vi "校准设置页.vi"() -> ()   [LabVIEW 2016, in "斯坦道总氮V2.lvlib"]
uses:
  <vilib>/regexp/Match Regular Expression.xnode
  <vilib>/ptbypt/NI_PtbyPt.lvlib
panel:
  in  "校准任务":bool
  in  "历史数据导入":T1(radio)
  out "刷新时间":string
  out "模型刷新":bool
  in  "校准按钮":T1(radio)
  in  "仪器写入":bool
  in  "辅助计算":bool
  in  "曲线模型":T2={"标液浓度1"=0.0, "测量吸光度1"=0.0, "样品1启用"=FALSE, "标液浓度2"=0.0, "测量吸光度2"=0.0, "样品2启用"=FALSE, "标液浓度3"=0.0, "测量吸光度3"=0.0, "样品3启用"=FALSE, "标液浓度4"=0.0, "测量吸光度4"=0.0, "样品4启用"=FALSE, "标液浓度5"=0.0, "测量吸光度5"=0.0, "样品5启用"=FALSE, "模型"=enum."线性", "精度"=4.0, "XY图"=[], "拟合公式"="", "r^2"=0.0, "标样一校准时间"=timestamp(0 s since 1904-01-01), "标样二校准时间"=timestamp(0 s since 1904-01-01), "标样三校准时间"=timestamp(0 s since 1904-01-01), "标样四校准时间"=timestamp(0 s since 1904-01-01), "标样五校准时间"=timestamp(0 s since 1904-01-01), "二次方程"={"c"=0.0, "x"=0.0, "x^2"=0.0}, "标定时间"=timestamp(0 s since 1904-01-01)} {"标定时间" format="%<%y/%m/%d %H:%M:%S>T"; "标样五校准时间" format="%<%y/%m/%d %H:%M:%S>T"; "标样四校准时间" format="%<%y/%m/%d %H:%M:%S>T"; "标样三校准时间" format="%<%y/%m/%d %H:%M:%S>T"; "标样二校准时间" format="%<%y/%m/%d %H:%M:%S>T"; "标样一校准时间" format="%<%y/%m/%d %H:%M:%S>T"; "r^2" format="%.7f"; "测量吸光度5" format="%#.6f"; "测量吸光度4" format="%#.6f"; "测量吸光度3" format="%#.6f"; "测量吸光度2" format="%#.6f"; "测量吸光度1" format="%#.6f"}
  in  "测量模式":enum16{"跨度核查", "水样测量", "零点核查", "标样核查", "加标回收"}(ring)
  in  "参数下拉列表":u16(ring)
  in  "量程下拉列表":enum16{"低量程", "高量程"}(ring)
  # "校准时间"
  # "标液浓度"
  # "吸光值"
  # "标样一"
  # "标样二"
  # "标样三"
  # "零点"
  # "跨度"
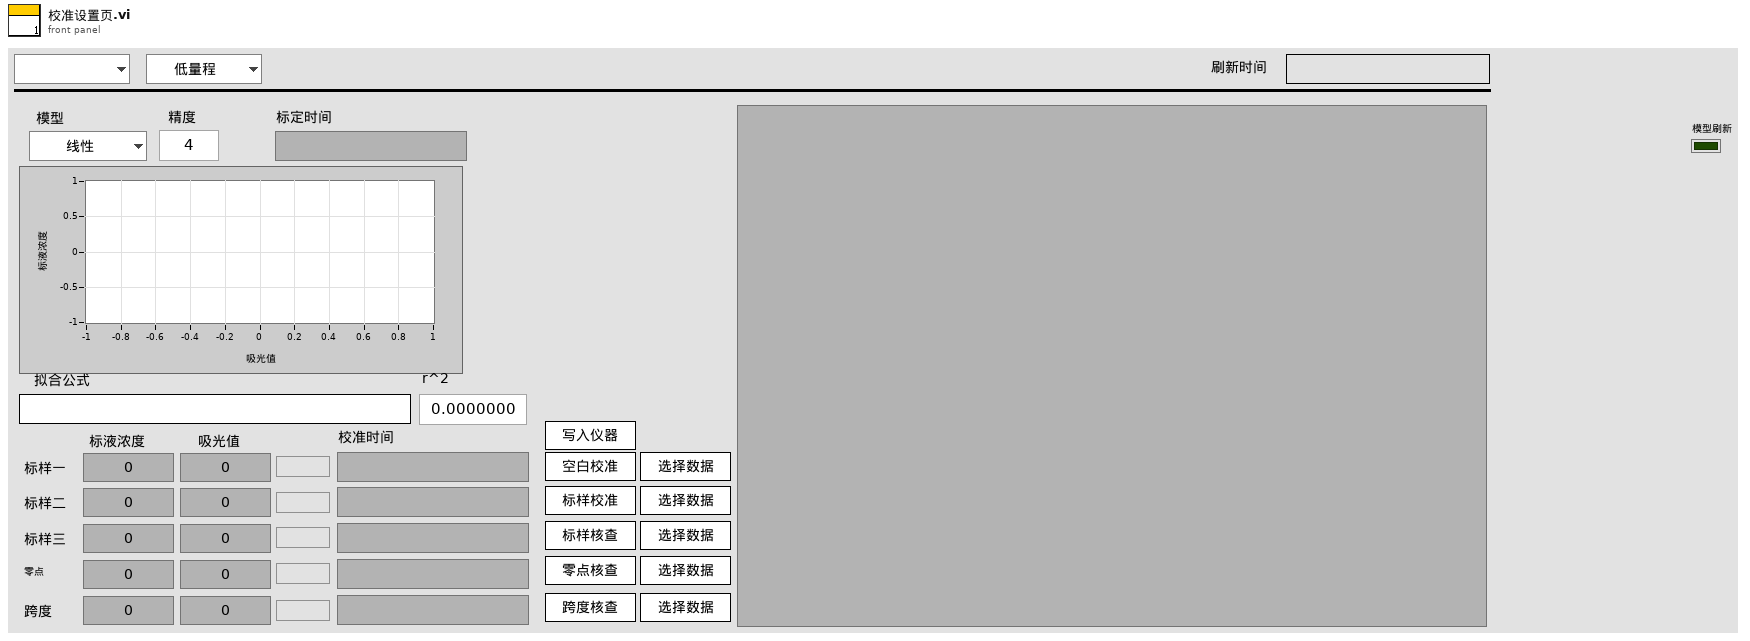
[diagram p1: front panel]
types:
  T1 = enum32{"未选择", "空白校准", "标样校准", "标样核查", "零点核查", "跨度核查"}
  T2 = cluster{"标液浓度1":dbl, "测量吸光度1":dbl, "样品1启用":bool, "标液浓度2":dbl, "测量吸光度2":dbl, "样品2启用":bool, "标液浓度3":dbl, "测量吸光度3":dbl, "样品3启用":bool, "标液浓度4":dbl, "测量吸光度4":dbl, "样品4启用":bool, "标液浓度5":dbl, "测量吸光度5":dbl, "样品5启用":bool, "模型":enum32{"线性", "多项式"}, "精度":dbl, "XY图":cluster{"X Values":dbl[], "Y Values":dbl[]}[], "拟合公式":string, "r^2":dbl, "标样一校准时间":timestamp, "标样二校准时间":timestamp, "标样三校准时间":timestamp, "标样四校准时间":timestamp, "标样五校准时间":timestamp, "二次方程":cluster{"c":dbl, "x":dbl, "x^2":dbl}, "标定时间":timestamp}
  T3 = typedef "斯坦道总氮V2.lvlib/校准任务.ctl" = cluster{"id":u16, "任务类型":enum16{"未选择", "空白校准", "标样校准", "标样核查", "零点核查", "跨度核查"}, "量程下拉列表":enum16{"低量程", "高量程"}, "状态":enum16{"已执行", "待执行", "执行中", "停止"}, "标液浓度":dbl, "吸光值":dbl, "校准时间":timestamp}
  T4 = enum8{"Enabled", "Disabled", "Disabled and Grayed Out"}
  T5 = enum16{"跨度核查", "水样测量", "零点核查", "标样核查", "加标回收", "快捷测试", "空白校准", "标样校准"}
  T6 = typedef "LVStringsAndValuesArrayTypeDef_U16.ctl" = cluster{"String":string, "Value":u16}[]
  T7 = cluster{"标液浓度1":dbl, "测量吸光度1":dbl, "样品1启用":bool, "标液浓度2":dbl, "测量吸光度2":dbl, "样品2启用":bool, "标液浓度3":dbl, "测量吸光度3":dbl, "样品3启用":bool, "标液浓度4":dbl, "测量吸光度4":dbl, "样品4启用":bool, "标液浓度5":dbl, "测量吸光度5":dbl, "样品5启用":bool, "模型":enum32{"线性", "多项式"}, "精度":dbl, "XY图":cluster{"X Values":dbl[], "Y Values":dbl[]}[], "拟合公式":string, "r^2":dbl, "标样一校准时间":timestamp, "标样二校准时间":timestamp, "标样三校准时间":timestamp, "标样四校准时间":timestamp, "标样五校准时间":timestamp, "二次方程":cluster{"c":dbl, "x":dbl, "x^2":dbl}, "标定时间":timestamp}[]
  T8 = cluster{"时间":timestamp, "标液值":dbl, "检测值":dbl, "吸光值":dbl}
  T9 = enum32{"Bad", "Idle", "Run top level", "Running"}
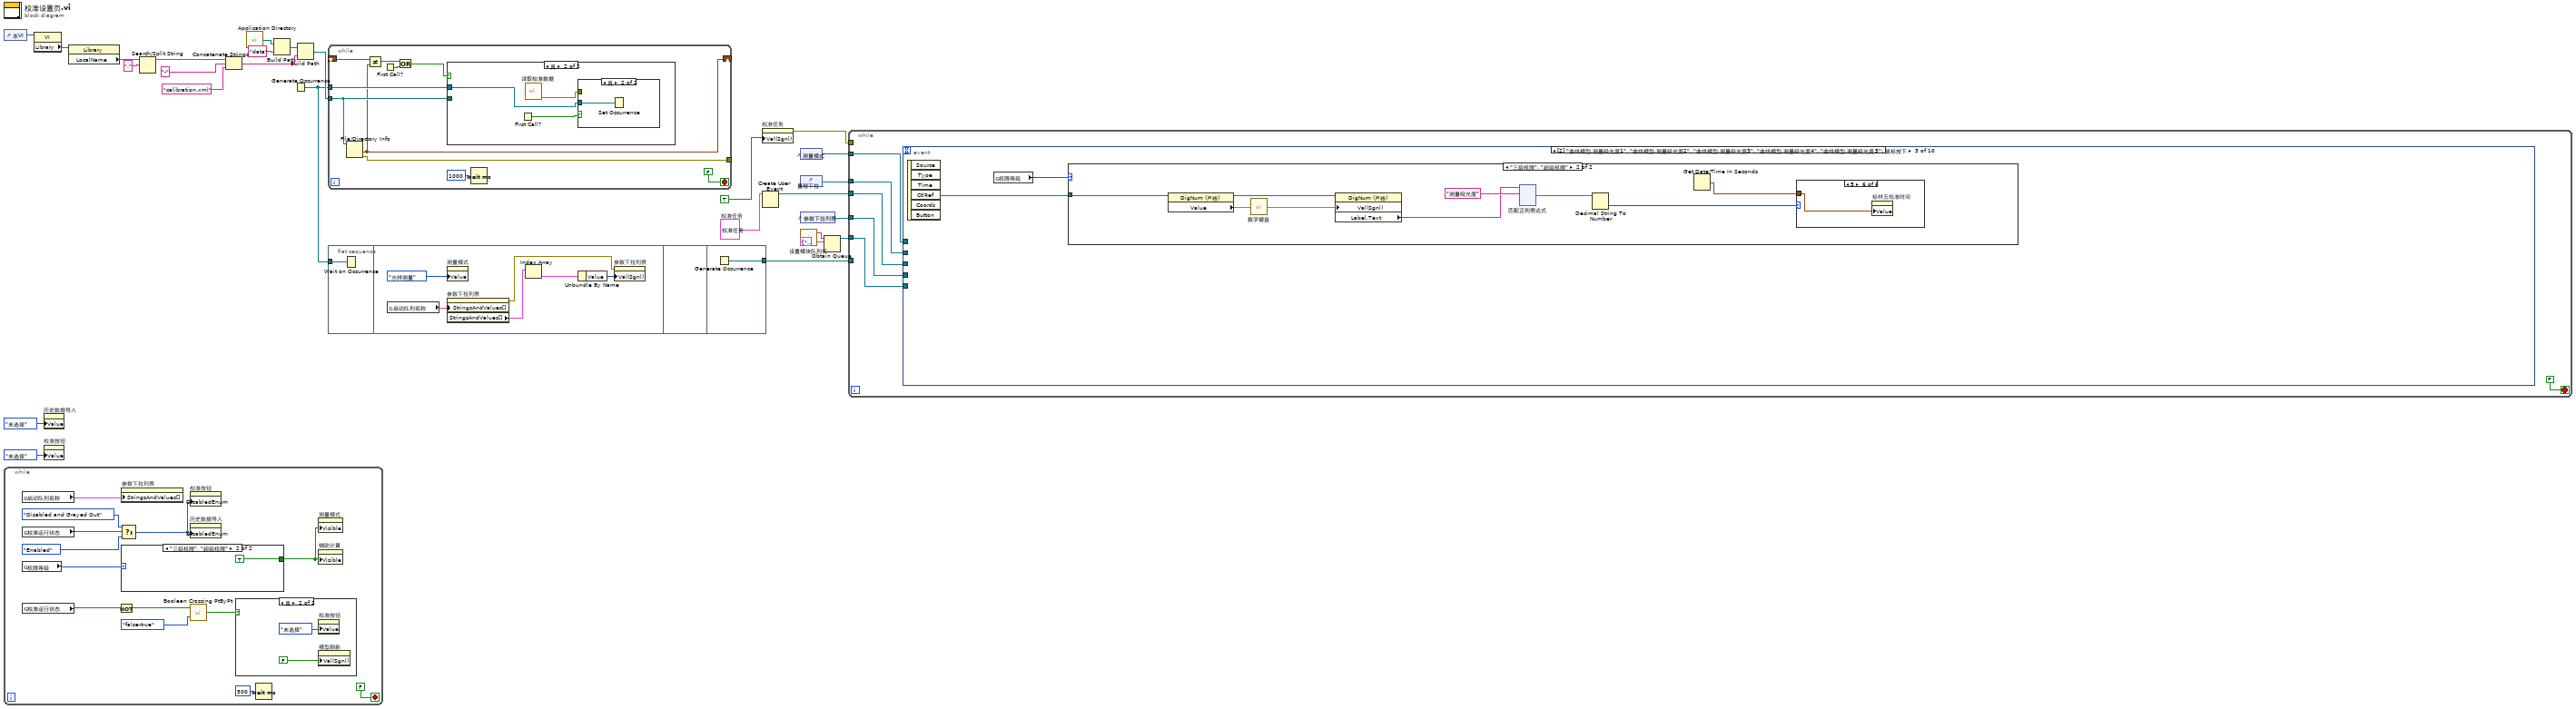
[diagram p0: block diagram]
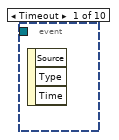
[diagram p4: hidden frame]
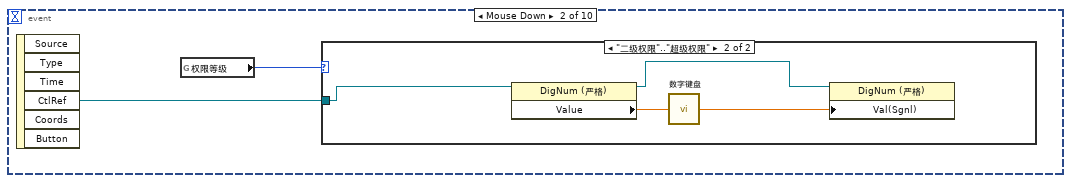
[diagram p5: hidden frame]
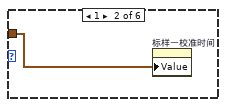
[diagram p9: hidden frame]
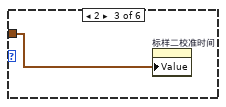
[diagram p10: hidden frame]
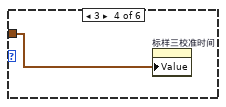
[diagram p11: hidden frame]
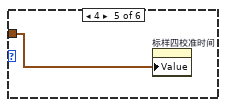
[diagram p12: hidden frame]
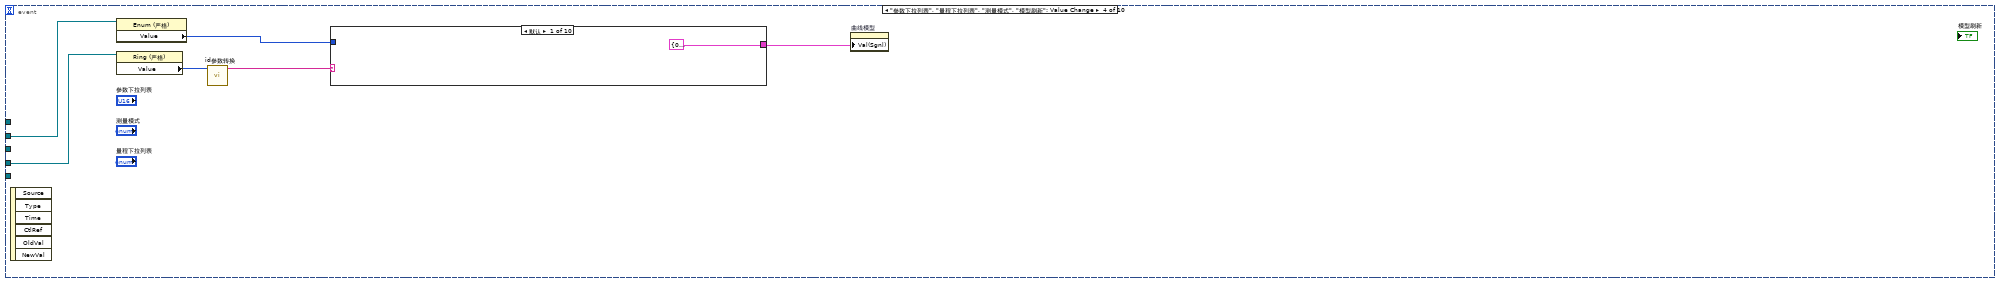
[diagram p13: hidden frame]
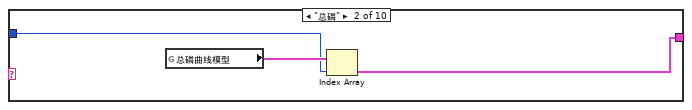
[diagram p14: hidden frame]
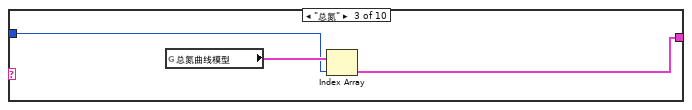
[diagram p15: hidden frame]
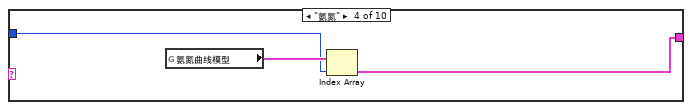
[diagram p16: hidden frame]
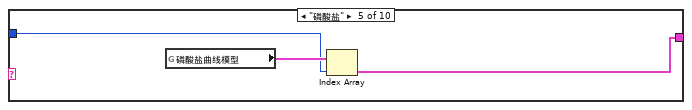
[diagram p17: hidden frame]
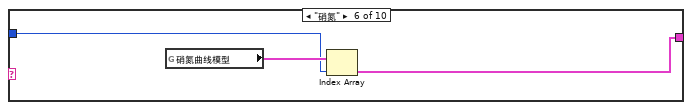
[diagram p18: hidden frame]
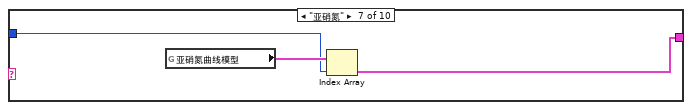
[diagram p19: hidden frame]
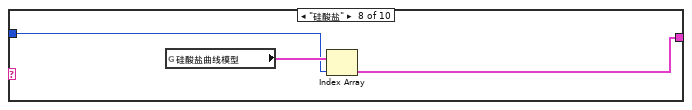
[diagram p20: hidden frame]
diagram:
  w3 = T3 {"id"=1, "任务类型"=enum."未选择", "量程下拉列表"=enum."低量程", "状态"=enum."已执行", "标液浓度"=0.0, "吸光值"=0.0, "校准时间"=timestamp(0 s since 1904-01-01)}  # 校准任务
  n1 = control-ref of="本VI"() -> (w14:refnum<vi>)
  n2 = while {
    stop <- FALSE stop-if-true
    n3 = global read "总磷总氮断电保存全局变量.vi" "启动队列名称"() -> (w34:cluster{"String":string, "Value":u16}[])
    n4 = global read "VAR总磷总氮全局变量.vi" "校准运行状态"() -> (w31:bool)
    n5 = global read "VAR总磷总氮全局变量.vi" "权限等级"() -> (w37:enum16{"一级权限", "二级权限", "三级权限", "超级权限"})
    n6 = global read "VAR总磷总氮全局变量.vi" "校准运行状态"() -> (w33:bool)
    n7 = Not(x=w33) -> (.not. x?=w32:bool)
    n8 = Select(t=T4."Disabled and Grayed Out" ("禁用"), s=w31, f=T4."Enabled" ("禁用")) -> (s? t:f=w29:T4)
    n9 = property on="参数下拉列表" class="Ring (严格)"("StringsAndValues[]"=w34) -> ()  [unwired: 2 in, 2 out]
    n10 = case shown="\"三级权限\", \"超级权限\"" w37 {
      tunnel: [_ TRUE ("可见")] -> w27
      frame "一级权限", Default {
        n11 = property on="测量模式" class="Enum (严格)"("Value"=T5."水样测量" ("测量模式")) -> ()  [unwired: 2 in, 2 out]
      }
      frame "三级权限", "超级权限" {
      }
    }
    n12 = property on="校准按钮" class="RadioBtnsControl (严格)"("DisabledEnum"=w29) -> ()  [unwired: 2 in, 2 out]
    n13 = property on="历史数据导入" class="RadioBtnsControl (严格)"("DisabledEnum"=w29) -> ()  [unwired: 2 in, 2 out]
    n14 = call <vilib>:"Boolean Crossing PtByPt.vi"("direction"=enum16{"either", "false-true", "true-false"}."false-true", "input"=w32) -> ("crossing"=w35:bool)  [unwired: 1 in]
    n15 = case shown="真" w35 {
      frame False {
      }
      frame True {
        n16 = property on="校准按钮" class="RadioBtnsControl (严格)"("Value"=T1."未选择" ("校准按钮")) -> ()  [unwired: 2 in, 2 out]
        n17 = property on="模型刷新" class="Bool (严格)"("Val(Sgnl)"=FALSE ("值(信号)")) -> ()  [unwired: 2 in, 2 out]
      }
    }
    n18 = Wait (ms)(milliseconds to wait=u32 500 ("等待时间（毫秒）")) -> ()  [unwired: 1 out]
    n19 = property on="测量模式" class="Enum (严格)"("Visible"=w27) -> ()  [unwired: 2 in, 2 out]
    n20 = property on="辅助计算" class="Bool"("Visible"=w27) -> ()  [unwired: 2 in, 2 out]
  }
  n21 = property class="VI"(reference=w14) -> ("Library"=w15:refnum<vi>)  [unwired: 1 in, 2 out]
  n22 = property on="历史数据导入" class="RadioBtnsControl (严格)"("Value"=T1."未选择" ("历史数据导入")) -> ()  [unwired: 2 in, 2 out]
  n23 = property on="校准按钮" class="RadioBtnsControl (严格)"("Value"=T1."未选择" ("校准按钮")) -> ()  [unwired: 2 in, 2 out]
  n24 = property class="Library"(reference=w15) -> ("LocalName"=w12:string)  [unwired: 1 in, 2 out]
  n25 = Search/Split String(string=w12, search string/char (-)="." ("搜索字符串/字符(-)")) -> (substring before match=w10:string)  [unwired: 1 in, 2 out]
  n26 = Concatenate Strings(w10, "-" ("字符串"), "calibration.xml" ("名称或相对路径")) -> (w7:string)
  n27 = call <vilib>:"Application Directory.vi"() -> ("Application Directory"=w16:path)
  n28 = Build Path(base path=w16, name or relative path="data" ("名称或相对路径")) -> (appended path=w13:path)
  n29 = Generate Occurrence() -> (w5:refnum<k4>)
  n30 = Build Path(base path=w13, name or relative path=w7) -> (appended path=w6:path)
  n31 = while {
    shift-right: [w44] -> _
    shift-left: _ -> [w52]
    tunnel: w6 -> [w50]
    tunnel: [w48] -> _
    tunnel: w5 -> [w47]
    stop <- FALSE stop-if-true
    n32 = File/Directory Info(path=w50) -> (last mod=w44:timestamp, error out=w48:errorcluster)  [unwired: 1 in, 5 out]
    n33 = Not Equal?(x=w52, y=w44) -> (x != y?=w51:bool)
    n34 = First Call?() -> (First Call?: T/F=w45:bool)
    n35 = Or(x=w51, y=w45) -> (x .or. y?=w46:bool)
    n36 = case shown="真" w46 {
      tunnel: w50 -> [_ _]
      tunnel: w47 -> [_ w56]
      frame False {
      }
      frame True {
        n37 = First Call?() -> (First Call?: T/F=w54:bool)
        n38 = call "读取校准数据.vi"() -> ("错误输出"=w55:errorcluster)  [unwired: 11 in]
        n39 = case shown="真" w54 {
          tunnel: w56 -> [_ w57]
          tunnel: w55 -> [_ _]
          frame False {
          }
          frame True {
            n40 = Set Occurrence(w57) -> ()
          }
        }
      }
    }
    n41 = Wait (ms)(milliseconds to wait=u32 1000 ("等待时间（毫秒）")) -> ()  [unwired: 1 out]
  }
  n42 = flat-sequence {
    tunnel: w5 -> [w58]
    tunnel: [w65] -> w26
    frame #0 {
      n43 = Wait on Occurrence(2:w58) -> ()  [unwired: 2 in, 1 out]
    }
    frame #1 {
      n44 = global read "总磷总氮断电保存全局变量.vi" "启动队列名称"() -> (w60:cluster{"String":string, "Value":u16}[])
      n45 = property on="测量模式" class="Enum (严格)"("Value"=T5."水样测量" ("测量模式")) -> ()  [unwired: 2 in, 2 out]
      n46 = property on="参数下拉列表" class="Ring (严格)"("StringsAndValues[]"=w60) -> (error out=w63:errorcluster, "StringsAndValues[]"=w61:T6)  [unwired: 2 in, 1 out]
      n47 = Index Array(array=w61) -> (element=w62:cluster{"String":string, "Value":u16})  [unwired: 1 in]
      n48 = Unbundle By Name(w62) -> ("Value"=w64:u16)
      n49 = property on="参数下拉列表" class="Ring (严格)"(error in=w63, "Val(Sgnl)"=w64) -> ()  [unwired: 1 in, 2 out]
    }
    frame #2 {
    }
    frame #3 {
      n50 = Generate Occurrence() -> (w65:refnum<k4>)
    }
  }
  n51 = property on="校准任务" class="Bool (严格)"("Val(Sgnl)"=TRUE ("值(信号)")) -> (error out=w2:errorcluster)  [unwired: 2 in, 1 out]
  n52 = Create User Event(user event datatype=w3) -> (user event=w4:refnum<user-event>)  [unwired: 1 in, 1 out]
  n53 = control-ref of="测量模式"() -> (w20:refnum<vi>)
  n54 = control-ref of="量程下拉列表"() -> (w19:refnum<vi>)
  n55 = control-ref of="参数下拉列表"() -> (w21:refnum<vi>)
  n56 = call "设置模块队列名.vi"() -> ("Msg"=w24:string)  [unwired: 5 in]
  n57 = Obtain Queue(name (unnamed)=w24, element data type=cluster{"命令":string, "data":variant} {"命令"="", "data"=variant}) -> (queue out=w23:refnum<queue>)  [unwired: 3 in, 2 out]
  n58 = while {
    tunnel: w26 -> [_]
    tunnel: w21 -> [w70]
    tunnel: w20 -> [w69]
    tunnel: w19 -> [w68]
    tunnel: w23 -> [w67]
    tunnel: w4 -> [w66]
    tunnel: w2 -> [_]
    stop <- FALSE stop-if-true
    n59 = event shown="[2] \"曲线模型.测量吸光度1\", \"曲线模型.测量吸光度2\", \"曲线模型.测量吸光度3\", \"曲线模型.测量吸光度4\", \"曲线模型.测量吸光度5\": 鼠标按下" {
      selector: _ -> [_ _ _ _ _ _ _ _ _ _]
      dyn-events: _ -> [_ _ _ _ _ _ _ _ _ _]
      timeout: _ -> [_ _ _ _ _ _ _ _ _ _]
      tunnel: w70 -> [_ _ _ w212 _ w267 w312 w366 w394 _]
      tunnel: w69 -> [_ _ _ _ _ w265 _ w361 w389 _]
      tunnel: w68 -> [_ _ _ w210 _ w263 w310 w365 w393 _]
      tunnel: w67 -> [_ _ _ _ _ _ _ w367 w395 _]
      tunnel: w66 -> [_ _ _ _ _ _ _ w360 w388 w417]
      event Timeout {
        n60 = event-data() -> ()  [unwired: 1 in, 3 out]
      }
      event "曲线模型.标液浓度1", "曲线模型.标液浓度2", "曲线模型.标液浓度3", "曲线模型.标液浓度4", "曲线模型.标液浓度5", "曲线模型.精度": Mouse Down {
        n61 = event-data() -> ("CtlRef"=w73:refnum<vi>)  [unwired: 1 in, 5 out]
        n62 = global read "VAR总磷总氮全局变量.vi" "权限等级"() -> (w72:enum16{"一级权限", "二级权限", "三级权限", "超级权限"})
        n63 = case shown="\"二级权限\"..\"超级权限\"" w72 {
          tunnel: w73 -> [_ w77]
          frame "一级权限", Default {
          }
          frame "二级权限".."超级权限" {
            n64 = property class="DigNum (严格)"(reference=w77) -> (reference out=w75:refnum<vi>, "Value"=w76:dbl)  [unwired: 1 in, 1 out]
            n65 = call "数字键盘.vi"("OldNumber"=w76) -> ("NewNumber"=w74:dbl)
            n66 = property class="DigNum (严格)"(reference=w75, "Val(Sgnl)"=w74) -> ()  [unwired: 1 in, 2 out]
          }
        }
      }
      event "曲线模型.测量吸光度1", "曲线模型.测量吸光度2", "曲线模型.测量吸光度3", "曲线模型.测量吸光度4", "曲线模型.测量吸光度5": Mouse Down {
        n67 = event-data() -> ("CtlRef"=w79:refnum<vi>)  [unwired: 1 in, 5 out]
        n68 = global read "VAR总磷总氮全局变量.vi" "权限等级"() -> (w78:enum16{"一级权限", "二级权限", "三级权限", "超级权限"})
        n69 = case shown="\"三级权限\", \"超级权限\"" w78 {
          tunnel: w79 -> [_ w88]
          frame "一级权限", Default {
          }
          frame "三级权限", "超级权限" {
            n70 = property class="DigNum (严格)"(reference=w88) -> (reference out=w86:refnum<vi>, "Value"=w87:dbl)  [unwired: 1 in, 1 out]
            n71 = call "数字键盘.vi"("OldNumber"=w87) -> ("NewNumber"=w85:dbl)
            n72 = property class="DigNum (严格)"(reference=w86, "Val(Sgnl)"=w85) -> ("Label.Text"=w80:string)  [unwired: 1 in, 2 out]
            n73 = xnode "匹配正则表达式"("输入字符串"=w80, "正则表达式"="测量吸光度" ("搜索字符串/字符(-)")) -> ("匹配之后"=w83:string)  [unwired: 4 in, 4 out]
            n74 = Decimal String To Number(string=w83) -> (number=w82:i32)  [unwired: 2 in, 1 out]
            n75 = Get Date/Time In Seconds() -> (seconds since 1Jan1904=w81:timestamp)
            n76 = case shown="5" w82 {
              tunnel: w81 -> [_ w89 w90 w91 w92 w93]
              frame 0, Default {
              }
              frame 1 {
                n77 = property on="标样一校准时间" class="AbsTime (严格)"("Value"=w89) -> ()  [unwired: 2 in, 2 out]
              }
              frame 2 {
                n78 = property on="标样二校准时间" class="AbsTime (严格)"("Value"=w90) -> ()  [unwired: 2 in, 2 out]
              }
              frame 3 {
                n79 = property on="标样三校准时间" class="AbsTime (严格)"("Value"=w91) -> ()  [unwired: 2 in, 2 out]
              }
              frame 4 {
                n80 = property on="标样四校准时间" class="AbsTime (严格)"("Value"=w92) -> ()  [unwired: 2 in, 2 out]
              }
              frame 5 {
                n81 = property on="标样五校准时间" class="AbsTime (严格)"("Value"=w93) -> ()  [unwired: 2 in, 2 out]
              }
            }
          }
        }
      }
      event "参数下拉列表", "量程下拉列表", "测量模式", "模型刷新": Value Change {
        n82 = event-data() -> ()  [unwired: 1 in, 6 out]
        n83 = property class="Enum (严格)"(reference=w210) -> ("Value"=w208:enum16{"低量程", "高量程"})  [unwired: 1 in, 2 out]
        n84 = property class="Ring (严格)"(reference=w212) -> ("Value"=w213:u16)  [unwired: 1 in, 2 out]
        n85 = call "id参数转换.vi"("id"=w213) -> ("table输出"=w211:string)  [unwired: 9 in, 1 out]
        n86 = case shown="默认" w211 {
          tunnel: w208 -> [_ w215 w218 w221 w224 w227 w230 w233 w236 w239]
          tunnel: [T2 {"标液浓度1"=0.0, "测量吸光度1"=0.0, "样品1启用"=FALSE, "标液浓度2"=0.0, "测量吸光度2"=0.0, "样品2启用"=FALSE, "标液浓度3"=0.0, "测量吸光度3"=0.0, "样品3启用"=FALSE, "标液浓度4"=0.0, "测量吸光度4"=0.0, "样品4启用"=FALSE, "标液浓度5"=0.0, "测量吸光度5"=0.0, "样品5启用"=FALSE, "模型"=enum."线性", "精度"=0.0, "XY图"=[], "拟合公式"="", "r^2"=0.0, "标样一校准时间"=timestamp(0 s since 1904-01-01), "标样二校准时间"=timestamp(0 s since 1904-01-01), "标样三校准时间"=timestamp(0 s since 1904-01-01), "标样四校准时间"=timestamp(0 s since 1904-01-01), "标样五校准时间"=timestamp(0 s since 1904-01-01), "二次方程"={"c"=0.0, "x"=0.0, "x^2"=0.0}, "标定时间"=timestamp(0 s since 1904-01-01)} ("总磷曲线模型") w216 w219 w222 w225 w228 w231 w234 w237 w240] -> w209
          frame Default {
          }
          frame "总磷" {
            n87 = global read "校准数据全局变量.vi" "总磷曲线模型"() -> (w217:T7)
            n88 = Index Array(array=w217, index=w215) -> (element=w216:T2)
          }
          frame "总氮" {
            n89 = global read "校准数据全局变量.vi" "总氮曲线模型"() -> (w220:T7)
            n90 = Index Array(array=w220, index=w218) -> (element=w219:T2)
          }
          frame "氨氮" {
            n91 = global read "校准数据全局变量.vi" "氨氮曲线模型"() -> (w223:T7)
            n92 = Index Array(array=w223, index=w221) -> (element=w222:T2)
          }
          frame "磷酸盐" {
            n93 = global read "校准数据全局变量.vi" "磷酸盐曲线模型"() -> (w226:T7)
            n94 = Index Array(array=w226, index=w224) -> (element=w225:T2)
          }
          frame "硝氮" {
            n95 = global read "校准数据全局变量.vi" "硝氮曲线模型"() -> (w229:T7)
            n96 = Index Array(array=w229, index=w227) -> (element=w228:T2)
          }
          frame "亚硝氮" {
            n97 = global read "校准数据全局变量.vi" "亚硝氮曲线模型"() -> (w232:T7)
            n98 = Index Array(array=w232, index=w230) -> (element=w231:T2)
          }
          frame "硅酸盐" {
            n99 = global read "校准数据全局变量.vi" "硅酸盐曲线模型"() -> (w235:T7)
            n100 = Index Array(array=w235, index=w233) -> (element=w234:T2)
          }
          frame "硫化物" {
            n101 = global read "校准数据全局变量.vi" "硫化物曲线模型"() -> (w238:T7)
            n102 = Index Array(array=w238, index=w236) -> (element=w237:T2)
          }
          frame "CODcr" {
            n103 = global read "校准数据全局变量.vi" "CODcr曲线模型"() -> (w241:T7)
            n104 = Index Array(array=w241, index=w239) -> (element=w240:T2)
          }
        }
        n105 = property on="曲线模型" class="Clust (严格)"("Val(Sgnl)"=w209) -> ()  [unwired: 2 in, 2 out]
      }
      event "辅助计算": Value Change {
        n106 = event-data() -> ()  [unwired: 1 in, 6 out]
        n107 = Get Date/Time In Seconds() -> (seconds since 1Jan1904=w242:timestamp)
        n108 = call "吸光值辅助计算.vi"() -> ("X"=w243:dbl, "吸光值导出"=w244:u16)  [unwired: 10 in]
        n109 = case shown="4" w244 {
          tunnel: w243 -> [_ w246 w248 w250 w252 w254]
          tunnel: w242 -> [_ w245 w247 w249 w251 w253]
          frame 0, Default {
          }
          frame 1 {
            n110 = property on="标样一校准时间" class="AbsTime (严格)"("Val(Sgnl)"=w245) -> ()  [unwired: 2 in, 2 out]
            n111 = property on="测量吸光度1" class="DigNum (严格)"("Value"=w246) -> ()  [unwired: 2 in, 2 out]
          }
          frame 2 {
            n112 = property on="标样二校准时间" class="AbsTime (严格)"("Val(Sgnl)"=w247) -> ()  [unwired: 2 in, 2 out]
            n113 = property on="测量吸光度2" class="DigNum (严格)"("Value"=w248) -> ()  [unwired: 2 in, 2 out]
          }
          frame 3 {
            n114 = property on="标样三校准时间" class="AbsTime (严格)"("Val(Sgnl)"=w249) -> ()  [unwired: 2 in, 2 out]
            n115 = property on="测量吸光度3" class="DigNum (严格)"("Value"=w250) -> ()  [unwired: 2 in, 2 out]
          }
          frame 4 {
            n116 = property on="标样四校准时间" class="AbsTime (严格)"("Val(Sgnl)"=w251) -> ()  [unwired: 2 in, 2 out]
            n117 = property on="测量吸光度4" class="DigNum (严格)"("Value"=w252) -> ()  [unwired: 2 in, 2 out]
          }
          frame 5 {
            n118 = property on="标样五校准时间" class="AbsTime (严格)"("Val(Sgnl)"=w253) -> ()  [unwired: 2 in, 2 out]
            n119 = property on="测量吸光度5" class="DigNum (严格)"("Value"=w254) -> ()  [unwired: 2 in, 2 out]
          }
        }
      }
      event "仪器写入": Value Change {
        n120 = event-data() -> ()  [unwired: 1 in, 6 out]
        n121 = property class="Enum (严格)"(reference=w265) -> ("Value"=w264:enum16{"跨度核查", "水样测量", "零点核查", "标样核查", "加标回收"})  [unwired: 1 in, 2 out]
        n122 = property on="二次方程" class="Clust (严格)"() -> ("Value"=w256:cluster{"c":dbl, "x":dbl, "x^2":dbl})  [unwired: 2 in, 2 out]
        n123 = property class="Enum (严格)"(reference=w263) -> ("Value"=w262:enum16{"低量程", "高量程"})  [unwired: 1 in, 2 out]
        n124 = property class="Ring (严格)"(reference=w267) -> ("Value"=w266:u16)  [unwired: 1 in, 2 out]
        n125 = Unbundle By Name(w256) -> ("x^2"=w258:dbl, "x"=w259:dbl, "c"=w260:dbl)
        n126 = Bundle By Name(cluster=cluster{"X^2":dbl, "X":dbl, "b":dbl} {"X^2"=0.0, "X"=0.0, "b"=0.0} ("公式"), "X^2"=w258, "X"=w259, "b"=w260) -> (w255:cluster{"X^2":dbl, "X":dbl, "b":dbl})
        n127 = global read "VAR总磷总氮全局变量.vi" "权限等级"() -> (w261:enum16{"一级权限", "二级权限", "三级权限", "超级权限"})
        n128 = case shown="\"一级权限\", 默认" w261 {
          tunnel: w266 -> [w276 w308]
          tunnel: w264 -> [w275 w307]
          tunnel: w262 -> [w274 w306]
          tunnel: w255 -> [w268 w305]
          frame "一级权限", Default {
            n129 = Cluster To Array(cluster=w268) -> (array=w273:dbl[])
            n130 = Add Array Elements(numeric array=w273) -> (sum=w272:dbl)
            n131 = Equal To 0?(x=w272) -> (x = 0?=w270:bool)
            n132 = Not A Number/Path/Refnum?(number/path/refnum=w272) -> (NaN/Path/Refnum?=w271:bool)
            n133 = Or(x=w270, y=w271) -> (x .or. y?=w269:bool)
            n134 = case shown="假" w269 {
              tunnel: w276 -> [w282 _]
              tunnel: w275 -> [w281 _]
              tunnel: w274 -> [w280 _]
              tunnel: w268 -> [w277 _]
              frame False {
                n135 = Two Button Dialog(message="请再一次确认是否导入" ("消息")) -> (T button?=w278:bool)  [unwired: 2 in]
                n136 = case shown="真" w278 {
                  tunnel: w282 -> [_ w284]
                  tunnel: w281 -> [_ w290]
                  tunnel: w280 -> [_ w283]
                  tunnel: w277 -> [_ w285]
                  frame False {
                  }
                  frame True {
                    n137 = for {
                      N: 8 -> [_]
                      tunnel: w284 -> [w296]
                      tunnel: w290 -> [_]
                      tunnel: w283 -> [w295]
                      shift-right: [w294] -> w288
                      shift-left: errorcluster {"status"=FALSE, "code"=0, "source"=""} ("error out") -> [w291]
                      tunnel: w285 -> [w292]
                      i -> [w293]
                      n138 = call "公式写入.vi"("公式"=w292, "error in (no error)"=w291, "量程下拉列表"=w295, "测量模式"=w293, "参数下拉列表"=w296) -> ("error out"=w294:errorcluster)  [unwired: 6 in]
                    }
                    n139 = case shown="无错误" w288 {
                      tunnel: ["写入成功" "写入失败"] -> w289
                      tunnel: w284 -> [w300 _]
                      tunnel: w283 -> [w299 _]
                      frame No Error {
                        n140 = Get Date/Time In Seconds() -> (seconds since 1Jan1904=w301:timestamp)
                        n141 = property on="标定时间" class="AbsTime (严格)"("Val(Sgnl)"=w301) -> (error out=w297:errorcluster)  [unwired: 2 in, 1 out]
                        n142 = property on="曲线模型" class="Clust (严格)"(error in=w297) -> ("Value"=w298:T2)  [unwired: 1 in, 2 out]
                        n143 = call "校准记录.vi"("曲线模型"=w298, "量程"=w299, "校准参数"=w300) -> ()  [unwired: 8 in, 1 out]
                      }
                      frame Error {
                      }
                    }
                    n144 = One Button Dialog(message=w289) -> ()  [unwired: 1 in, 1 out]
                  }
                }
              }
              frame True {
                n145 = One Button Dialog(message="校准数据异常，请重新校准！" ("消息")) -> ()  [unwired: 1 in, 1 out]
              }
            }
          }
          frame "三级权限", "超级权限" {
            n146 = call "公式复合写入.vi"("公式"=w305, "量程下拉列表"=w306, "测量模式"=w307, "参数下拉列表"=w308) -> ()  [unwired: 8 in]
          }
        }
      }
      event "曲线模型": Value Change {
        n147 = event-data() -> ()  [unwired: 1 in, 6 out]
        n148 = flat-sequence {
          tunnel: [w317] -> w313
          tunnel: w312 -> [w317]
          tunnel: [w316] -> w311
          tunnel: w310 -> [w316]
          tunnel: w313 -> [w323]
          tunnel: w311 -> [w320]
          frame #0 {
            n149 = property on="曲线模型" class="Clust (严格)"() -> ("Value"=w315:T2)  [unwired: 2 in, 2 out]
            n150 = call "曲线模型计算.vi"("曲线模型"=w315) -> ("输出簇"=w314:T2)  [unwired: 10 in]
            n151 = property on="曲线模型" class="Clust (严格)"("Value"=w314) -> ()  [unwired: 2 in, 2 out]
          }
          frame #1 {
            n152 = property class="Enum (严格)"(reference=w320) -> ("Value"=w319:enum16{"低量程", "高量程"})  [unwired: 1 in, 2 out]
            n153 = property class="Ring (严格)"(reference=w323) -> ("Value"=w322:u16)  [unwired: 1 in, 2 out]
            n154 = call "id参数转换.vi"("id"=w322) -> ("table输出"=w321:string)  [unwired: 9 in, 1 out]
            n155 = property on="曲线模型" class="Clust (严格)"() -> ("Value"=w318:T2)  [unwired: 2 in, 2 out]
            n156 = case shown="\"总磷\"" w321 {
              tunnel: w318 -> [_ w325 w331 w334 w337 w341 w345 w349 w353 w358]
              tunnel: w319 -> [_ w324 w328 w332 w336 w340 w344 w348 w352 w356]
              frame Default {
              }
              frame "总磷" {
                n157 = global read "校准数据全局变量.vi" "总磷曲线模型"() -> (w326:T7)
                n158 = Replace Array Subset(array=w326, new element=w325, index=w324) -> (w327:T7)
                n159 = global write "校准数据全局变量.vi" "总磷曲线模型"(w327) -> ()
              }
              frame "总氮" {
                n160 = global read "校准数据全局变量.vi" "总氮曲线模型"() -> (w330:T7)
                n161 = Replace Array Subset(array=w330, new element=w331, index=w328) -> (w329:T7)
                n162 = global write "校准数据全局变量.vi" "总氮曲线模型"(w329) -> ()
              }
              frame "氨氮" {
                n163 = global read "校准数据全局变量.vi" "氨氮曲线模型"() -> (w335:T7)
                n164 = Replace Array Subset(array=w335, new element=w334, index=w332) -> (w333:T7)
                n165 = global write "校准数据全局变量.vi" "氨氮曲线模型"(w333) -> ()
              }
              frame "磷酸盐" {
                n166 = global read "校准数据全局变量.vi" "磷酸盐曲线模型"() -> (w339:T7)
                n167 = Replace Array Subset(array=w339, new element=w337, index=w336) -> (w338:T7)
                n168 = global write "校准数据全局变量.vi" "磷酸盐曲线模型"(w338) -> ()
              }
              frame "硝氮" {
                n169 = global read "校准数据全局变量.vi" "硝氮曲线模型"() -> (w343:T7)
                n170 = Replace Array Subset(array=w343, new element=w341, index=w340) -> (w342:T7)
                n171 = global write "校准数据全局变量.vi" "硝氮曲线模型"(w342) -> ()
              }
              frame "亚硝氮" {
                n172 = global read "校准数据全局变量.vi" "亚硝氮曲线模型"() -> (w347:T7)
                n173 = Replace Array Subset(array=w347, new element=w345, index=w344) -> (w346:T7)
                n174 = global write "校准数据全局变量.vi" "亚硝氮曲线模型"(w346) -> ()
              }
              frame "硅酸盐" {
                n175 = global read "校准数据全局变量.vi" "硅酸盐曲线模型"() -> (w351:T7)
                n176 = Replace Array Subset(array=w351, new element=w349, index=w348) -> (w350:T7)
                n177 = global write "校准数据全局变量.vi" "硅酸盐曲线模型"(w350) -> ()
              }
              frame "硫化物" {
                n178 = global read "校准数据全局变量.vi" "硫化物曲线模型"() -> (w355:T7)
                n179 = Replace Array Subset(array=w355, new element=w353, index=w352) -> (w354:T7)
                n180 = global write "校准数据全局变量.vi" "硫化物曲线模型"(w354) -> ()
              }
              frame "CODcr" {
                n181 = global read "校准数据全局变量.vi" "CODcr曲线模型"() -> (w359:T7)
                n182 = Replace Array Subset(array=w359, new element=w358, index=w356) -> (w357:T7)
                n183 = global write "校准数据全局变量.vi" "CODcr曲线模型"(w357) -> ()
              }
            }
          }
          frame #2 {
            n184 = call "校准数据写入配置文件.vi"() -> ()  [unwired: 11 in, 1 out]
          }
        }
        n185 = Format Date/Time String() -> (date/time string=→"刷新时间":string)  [unwired: 3 in]
      }
      event "校准按钮": Value Change {
        n186 = event-data() -> ("NewVal"=w362:T1)  [unwired: 1 in, 5 out]
        n187 = Not Equal?(x=w362, y=T1."未选择") -> (x != y?=w363:bool)
        n188 = case shown="真" w363 {
          tunnel: w367 -> [_ _]
          tunnel: w366 -> [_ w377]
          tunnel: w365 -> [_ w376]
          tunnel: w362 -> [_ w372]
          tunnel: w361 -> [_ _]
          tunnel: w360 -> [_ w375]
          frame False {
          }
          frame True {
            w369 = T3 {"id"=1, "任务类型"=enum."未选择", "量程下拉列表"=enum."低量程", "状态"=enum."待执行", "标液浓度"=0.0, "吸光值"=0.0, "校准时间"=timestamp(0 s since 1904-01-01)}  # 校准任务
            n189 = property class="Ring (严格)"(reference=w377) -> ("Value"=w374:u16)  [unwired: 1 in, 2 out]
            n190 = property class="Enum (严格)"(reference=w376) -> ("Value"=w373:enum16{"低量程", "高量程"})  [unwired: 1 in, 2 out]
            n191 = property on="曲线模型" class="Clust (严格)"() -> ("Value"=w371:T2)  [unwired: 2 in, 2 out]
            n192 = case shown="\"标样核查\"" w372 {
              tunnel: w371 -> [_ w379 w381 w383 w385 w387]
              tunnel: [_ w378 w380 w382 w384 w386] -> w370
              frame "未选择", Default {
              }
              frame "空白校准" {
                n193 = Unbundle By Name(w379) -> ("标液浓度1"=w378:dbl)
              }
              frame "标样校准" {
                n194 = Unbundle By Name(w381) -> ("标液浓度2"=w380:dbl)
              }
              frame "标样核查" {
                n195 = Unbundle By Name(w383) -> ("标液浓度3"=w382:dbl)
              }
              frame "零点核查" {
                n196 = Unbundle By Name(w385) -> ("标液浓度4"=w384:dbl)
              }
              frame "跨度核查" {
                n197 = Unbundle By Name(w387) -> ("标液浓度5"=w386:dbl)
              }
            }
            n198 = Bundle By Name(cluster=w369, "id"=w374, "任务类型"=w372, "量程下拉列表"=w373, "标液浓度"=w370) -> (w368:T3)
            n199 = Generate User Event(user event=w375, event data cluster=w368) -> ()  [unwired: 2 in, 2 out]
          }
        }
      }
      event "历史数据导入": Value Change {
        n200 = event-data() -> ("NewVal"=w390:T1)  [unwired: 1 in, 5 out]
        n201 = Not Equal?(x=w390, y=T1."未选择") -> (x != y?=w391:bool)
        n202 = case shown="真" w391 {
          tunnel: w395 -> [_ _]
          tunnel: w394 -> [_ w405]
          tunnel: w393 -> [_ w398]
          tunnel: w390 -> [_ w396]
          tunnel: w389 -> [_ _]
          tunnel: w388 -> [_ w400]
          frame False {
          }
          frame True {
            n203 = property class="Ring (严格)"(reference=w405) -> ("Value"=w399:u16)  [unwired: 1 in, 2 out]
            n204 = property class="Enum (严格)"(reference=w398) -> ("Value"=w397:enum16{"低量程", "高量程"})  [unwired: 1 in, 2 out]
            n205 = property on="历史数据导入" class="RadioBtnsControl (严格)"("Value"=T1."未选择" ("历史数据导入")) -> ()  [unwired: 2 in, 2 out]
            n206 = call "id参数转换.vi"("id"=w399) -> ("table输出"=w404:string)  [unwired: 9 in, 1 out]
            n207 = call "校准数据选择表.vi"("测量模式"=w396, "量程下拉列表"=w397, "table"=w404) -> ("布尔"=w403:bool, "输出"=w402:T8)  [unwired: 7 in]
            n208 = case shown="真" w403 {
              tunnel: w402 -> [_ w413]
              tunnel: w396 -> [_ w415]
              tunnel: w400 -> [_ w414]
              tunnel: w399 -> [_ w412]
              tunnel: w397 -> [_ w411]
              frame False {
              }
              frame True {
                w409 = T3 {"id"=1, "任务类型"=enum."未选择", "量程下拉列表"=enum."低量程", "状态"=enum."已执行", "标液浓度"=0.0, "吸光值"=0.0, "校准时间"=timestamp(0 s since 1904-01-01)}  # 校准任务
                n209 = Unbundle By Name(w413) -> ("标液值"=w406:dbl, "吸光值"=w407:dbl, "时间"=w408:timestamp)
                n210 = Bundle By Name(cluster=w409, "id"=w412, "任务类型"=w415, "量程下拉列表"=w411, "标液浓度"=w406, "吸光值"=w407, "校准时间"=w408) -> (w410:T3)
                n211 = Generate User Event(user event=w414, event data cluster=w410) -> ()  [unwired: 2 in, 2 out]
              }
            }
          }
        }
      }
      event "校准任务": Value Change {
        n212 = event-data() -> ("NewVal"=w416:bool)  [unwired: 1 in, 5 out]
        n213 = invoke on="子面板" class="SubPnl" method="Remove VI"() -> (error out=w418:errorcluster)  [unwired: 3 in, 2 out]
        n214 = case shown="真" w416 {
          tunnel: w418 -> [_ w425]
          tunnel: w417 -> [_ w422]
          frame False {
          }
          frame True {
            n215 = vi-ref "校准任务设置.vi"() -> (w424:refnum<vi>)
            n216 = property class="VI"(reference=w424) -> (reference out=w420:refnum<vi>, "Name"=w423:string, "Exec.State"=w421:T9)  [unwired: 1 in, 1 out]
            n217 = case shown="\"Idle\"" w421 {
              tunnel: w423 -> [_ w437]
              tunnel: w422 -> [_ w434]
              tunnel: [w426 w430] -> w419
              tunnel: w420 -> [w426 w430]
              frame "Bad", Default {
              }
              frame "Idle" {
                n218 = Open VI Reference(type specifier VI Refnum (for type only)=refnum<vi> refnum, vi path=w437, options=128 ("选项")) -> (vi reference=w435:refnum<vi>, error out=w432:errorcluster)  [unwired: 3 in]
                n219 = property on="模型" class="Enum (严格)"() -> ("Value"=w428:enum32{"线性", "多项式"})  [unwired: 2 in, 2 out]
                n220 = property on="精度" class="DigNum (严格)"() -> ("Value"=w427:dbl)  [unwired: 2 in, 2 out]
                n221 = call-by-ref "开始异步调用"(reference=w435, error in=w432, "精度"=w427, "模型"=w428, "用户事件"=w434) -> (reference out=w433:refnum<vi>, error out=w431:errorcluster)  [unwired: 9 in]
                n222 = Close Reference(reference=w433, error in (no error)=w431) -> ()  [unwired: 1 out]
              }
            }
            n223 = invoke on="子面板" class="SubPnl" method="Insert VI"(error in=w425, "VI Ref"=w419) -> ()  [unwired: 2 in, 4 out]
          }
        }
      }
    }
  }
